vi "open bitmap 24b 320x240.vi"(0 "path to BMP file":path) -> (4 "raw data":u16[][](array[numeric]), 8 "image ok":bool)   [LabVIEW 2010]
uses:
  <vilib>/picture/picture.llb/imagedata.ctl
panel:
  out "B 2":u8
  out "G 2":u8
  out "R 2":u8
  out "B":u8
  out "G":u8
  out "R":u8
  out "24-bit pixmap":u32[][](array[numeric]) format="%x"
  out "image data":T1
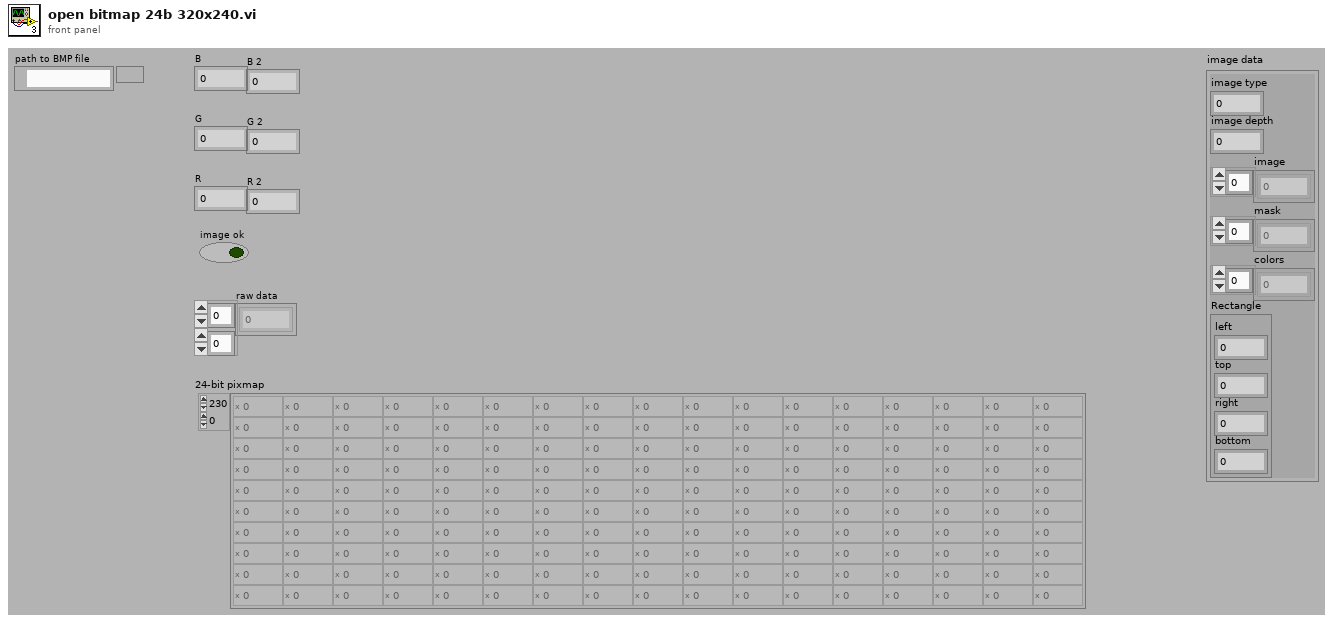
[diagram p1: front panel]
types:
  T1 = typedef "imagedata.ctl" = cluster{"image type":i32, "image depth":i32, "image":u8[], "mask":u8[], "colors":u32[], "Rectangle":cluster{"left":i16, "top":i16, "right":i16, "bottom":i16}}
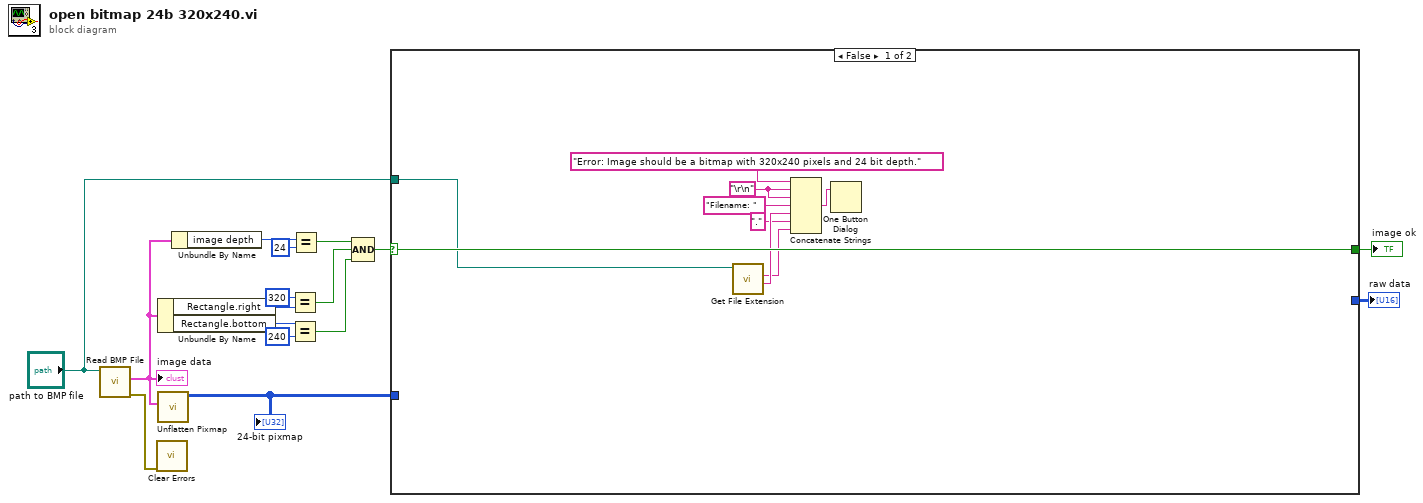
[diagram p0: block diagram]
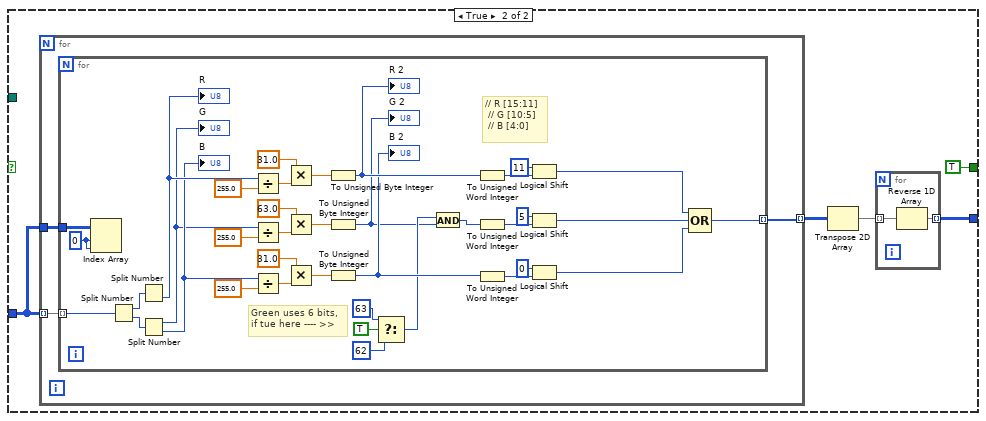
[diagram p2: hidden frame]
diagram:
  n1 = call <vilib>:"Read BMP File.vi"("path to BMP file"="path to BMP file") -> ("error out"=w16:errorcluster, "image data"=w6:T1)  [unwired: 8 in, 1 out]
  "image data" <- w6
  n2 = call <vilib>:"Clear Errors.vi"("error in (no error)"=w16) -> ()  [unwired: 6 in, 1 out]
  n3 = Unbundle By Name(w6) -> ("Rectangle.right"=w3:i16, "Rectangle.bottom"=w2:i16)
  n4 = call <vilib>:"Unflatten Pixmap.vi"("image data"=w6) -> ("24-bit pixmap"=w13:u32[][])  [unwired: 4 in, 6 out]
  "24-bit pixmap" <- w13
  n5 = Unbundle By Name(w6) -> ("image depth"=w7:i32)
  n6 = Equal?(x=i16 320, y=w3) -> (x = y?=w10:bool)
  n7 = Equal?(x=w2, y=i16 240) -> (x = y?=w11:bool)
  n8 = Equal?(x=w7, y=24) -> (x = y?=w9:bool)
  n9 = Compound Arithmetic op=AND(w9, w10, w11) -> (w12:bool)
  n10 = case shown="False" w12 {
    selector: w12 -> [w25 _]
    tunnel: w13 -> [_ w30]
    tunnel: [w25 TRUE] -> w14
    tunnel: [_ w27] -> w15
    tunnel: "path to BMP file" -> [w17 _]
    frame False {
      w22 = "\r\n"
      n11 = call <vilib>:"Get File Extension.vi"("file"=w17) -> ("filename without extension"=w20:string, "lowercase file extension"=w19:string)  [unwired: 7 in, 2 out]
      n12 = Concatenate Strings("Error: Image should be a bitmap with 320x240 pixels and 24 bit depth." ("message"), w22, w22, "Filename: " ("string"), w20, "." ("string"), w19) -> (w24:string)
      n13 = One Button Dialog(message=w24) -> ()  [unwired: 1 in, 1 out]
    }
    frame True {
      n14 = for {
        tunnel: w30 -> [w35] mode=indexing
        tunnel: w30 -> [w34]
        tunnel: [w33] -> w28 mode=indexing
        n15 = for {
          tunnel: w35 -> [w44] mode=indexing
          tunnel: w34 -> [w71]
          tunnel: [w39] -> w33 mode=indexing
          w70 = 0 ("index (row)")
          # "Green uses 6 bits,\nif tue here ---- >>"
          # "// R [15:11]\n\t// G [10:5]\n\t// B [4:0]"
          n16 = Index Array(array=w71, index (row)=w70, index (col)=w70) -> ()  [unwired: 1 out]
          n17 = Split Number(x=w44) -> (hi(x)=w73:u16, lo(x)=w72:u16)
          n18 = Split Number(x=w73) -> (lo(x)=w68:u8)  [unwired: 1 out]
          "R" <- w68
          n19 = Split Number(x=w72) -> (hi(x)=w55:u8, lo(x)=w56:u8)
          "G" <- w55
          "B" <- w56
          n20 = Divide(x=w68, y=255.0) -> (x/y=w67:dbl)
          n21 = Divide(x=w55, y=255.0) -> (x/y=w62:dbl)
          n22 = Divide(x=w56, y=255.0) -> (x/y=w59:dbl)
          n23 = Multiply(x=31.0, y=w67) -> (x*y=w65:dbl)
          n24 = Multiply(x=63.0, y=w62) -> (x*y=w64:dbl)
          n25 = Multiply(x=31.0, y=w59) -> (x*y=w57:dbl)
          n26 = To Unsigned Byte Integer(number=w65) -> (unsigned 8bit integer=w54:u8)
          "R 2" <- w54
          n27 = To Unsigned Byte Integer(number=w64) -> (unsigned 8bit integer=w37:u8)
          "G 2" <- w37
          n28 = To Unsigned Byte Integer(number=w57) -> (unsigned 8bit integer=w49:u8)
          "B 2" <- w49
          n29 = Select(t=u8 63 ("y"), s=TRUE, f=u8 62 ("y")) -> (s? t:f=w48:u8)
          n30 = And(x=w48, y=w37) -> (x .and. y?=w36:u8)
          n31 = To Unsigned Word Integer(number=w54) -> (unsigned 16bit integer=w53:u16)
          n32 = To Unsigned Word Integer(number=w36) -> (unsigned 16bit integer=w51:u16)
          n33 = To Unsigned Word Integer(number=w49) -> (unsigned 16bit integer=w50:u16)
          n34 = Logical Shift(y=i8 11, x=w53) -> (x << y=w41:u16)
          n35 = Logical Shift(y=i8 5, x=w51) -> (x << y=w38:u16)
          n36 = Logical Shift(y=i8 0, x=w50) -> (x << y=w40:u16)
          n37 = Compound Arithmetic op=OR(w41, w38, w40) -> (w39:u16)
        }
      }
      n38 = Transpose 2D Array(2D array=w28) -> (transposed array=w26:u16[][])
      n39 = for {
        tunnel: [w31] -> w27 mode=indexing
        tunnel: w26 -> [w32] mode=indexing
        n40 = Reverse 1D Array(array=w32) -> (reversed array=w31:u16[])
      }
    }
  }
  "raw data" <- w15
  "image ok" <- w14
